vi "Remove_unprintable_Char.vi"(1 "Input String":string="\u0000Hello Fred Bloggs\n\n\u0000") -> (0 "Output String":string)   [LabVIEW 2010]
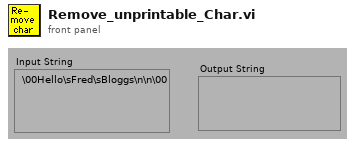
[diagram p1: front panel]
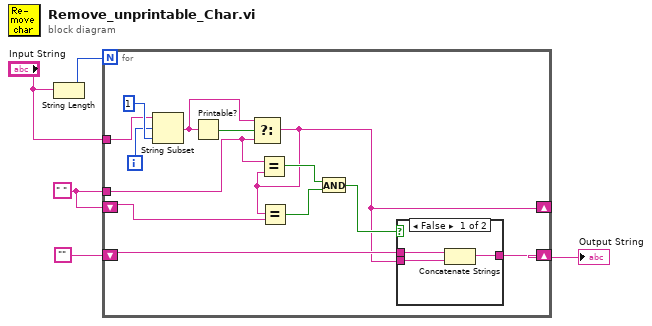
[diagram p0: block diagram]
diagram:
  w1 = " "
  n1 = String Length(string="Input String") -> (length=w5:i32)
  n2 = for {
    N: w5 -> [_]
    tunnel: "Input String" -> [w16]
    shift-right: [w14] -> w3
    shift-left: "" -> [w15]
    shift-right: [w6] -> _
    shift-left: w1 -> [w11]
    tunnel: w1 -> [w7]
    i -> [w17]
    n3 = String Subset(string=w16, offset (0)=w17, length (rest)=1 ("length")) -> (substring=w12:string)
    n4 = Printable?(1:w12) -> (0:w13:bool)
    n5 = Select(t=w12, s=w13, f=w7) -> (s? t:f=w6:string)
    n6 = Equal?(x=w7, y=w6) -> (x = y?=w10:bool)
    n7 = Equal?(x=w6, y=w11) -> (x = y?=w9:bool)
    n8 = And(x=w10, y=w9) -> (x .and. y?=w8:bool)
    n9 = case shown="False" w8 {
      tunnel: w15 -> [w21 w22]
      tunnel: [w20 w22] -> w14
      tunnel: w6 -> [w19 _]
      frame False {
        n10 = Concatenate Strings(w21, w19) -> (w20:string)
      }
      frame True {
      }
    }
  }
  "Output String" <- w3
